vi "Main Page GUID.vi"() -> (3 "Data Sharing Framework":string="37c56d03-17da-482b-8988-568955beadf2")   [LabVIEW 2017, in "Data Sharing Framework System Explorer.lvlib"]
uses:
  Data Sharing Framework System Explorer.lvlib
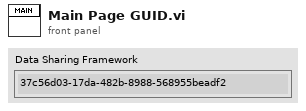
[diagram p1: front panel]
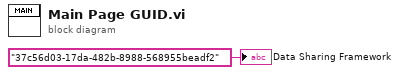
[diagram p0: block diagram]
diagram:
  "Data Sharing Framework" <- "37c56d03-17da-482b-8988-568955beadf2" ("Data Sharing Framework")
